vi "FGA Unfeed Watchdog.vi"(0 "Watchdog Dish Label":T1) -> ()   [LabVIEW 2009]
uses:
  UI Comm/Watchdog Dish Labels.ctl
  Actions for FG's.ctl
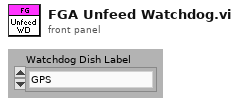
[diagram p1: front panel]
types:
  T1 = typedef "Watchdog Dish Labels.ctl" = enum16{"GPS", "SICK", "Compass", "Cameras", "Motor Controller", "Debug", "RC Receiver"}
  T2 = typedef "Actions for FG's.ctl" = enum16{"Read", "Write"}
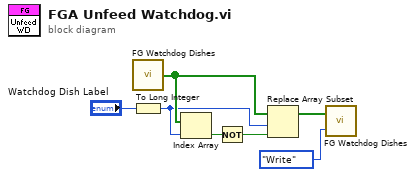
[diagram p0: block diagram]
diagram:
  n1 = call "FG Watchdog Dishes.vi"() -> ("Watchdog dishes out"=w5:bool[])  [unwired: 2 in]
  n2 = To Long Integer(number="Watchdog Dish Label") -> (32bit integer=w4:i32)
  n3 = Index Array(array=w5, index=w4) -> (element=w3:bool)
  n4 = Not(x=w3) -> (.not. x?=w2:bool)
  n5 = Replace Array Subset(array=w5, new element=w2, index=w4) -> (w1:bool[])
  n6 = call "FG Watchdog Dishes.vi"("FG Action (Read)"=Actions_for_FG's."Write", "Watchdog dishes in"=w1) -> ()  [unwired: 1 out]
